vi "HW Configurations.vi"() -> ()   [LabVIEW 2014]
uses:
  General/Controls/Translation Stage Types.ctl
panel:
  in  "Z Table Stage":T1 caption="Device Type"
  in  "Y Table Stage":T1=enum."Thorlabs LTS" caption="Device Type"
  in  "X Table Stage":T1=enum."Thorlabs LTS" caption="Device Type"
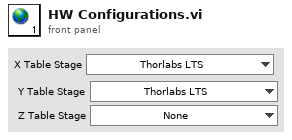
[diagram p1: front panel]
types:
  T1 = typedef "Translation Stage Types.ctl" = enum16{"None", "Thorlabs LTS", "Thorlabs MLJ"}
diagram:
